vi "Write CalPath.vi"(8 "error in (no error)":errorcluster, 10 "CalPath":path=path "c:/exscalabar/cals", 11 "Calibration Actor in":refnum<class "Calibration Actor.lvclass">) -> (0 "error out":errorcluster, 3 "Calibration Actor out":refnum<class "Calibration Actor.lvclass">)   [LabVIEW 2014, in "Calibration.lvlib" / "Calibration Actor.lvclass"]
uses:
  Calibration Actor.lvclass
  Calibration Actor.lvclass/Calibration Actor.ctl
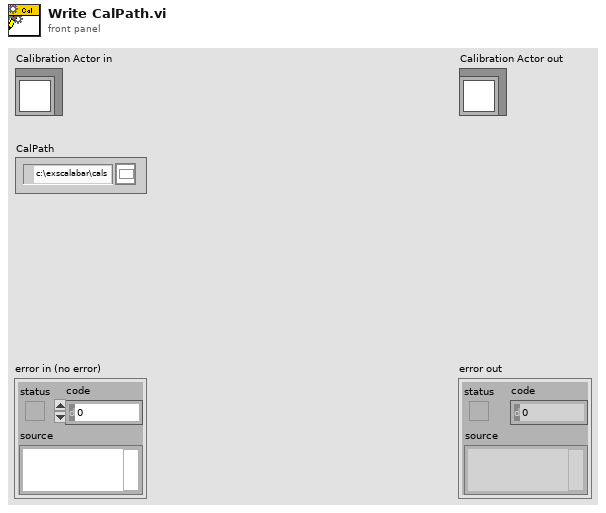
[diagram p1: front panel]
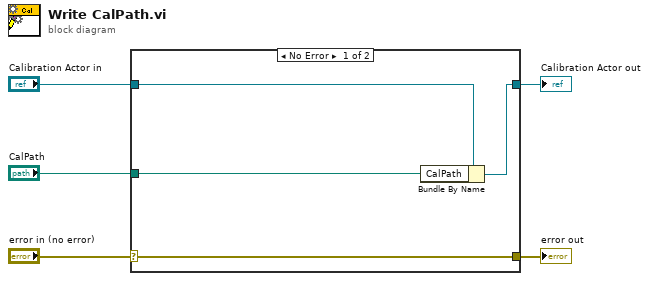
[diagram p0: block diagram]
diagram:
  n1 = case shown="No Error" "error in (no error)" {
    selector: "error in (no error)" -> [w9 w10]
    tunnel: [w9 w10] -> w4
    tunnel: [w7 w11] -> w2
    tunnel: "Calibration Actor in" -> [w8 w11]
    tunnel: "CalPath" -> [w6 _]
    frame No Error {
      n2 = Bundle By Name(cluster=w8, "CalPath"=w6) -> (w7:refnum<class "Calibration Actor.lvclass">)
    }
    frame Error {
    }
  }
  "error out" <- w4
  "Calibration Actor out" <- w2
